vi "MOV and qTAV.vi"(0 "System no.":i32=1 min=1 max=4 step=1, 1 "Board":i32=1 min=1 max=5 step=1, 2 "Axes to move":string[](array[string]), 3 "Position values":dbl[](array[numeric]) format="%.6f", 4 "No.of digits":i16=4, 5 "error in":errorcluster, 7 "Polling\nCycle time, ms":u32=1, 9 "Wait before\nTAV?, ms":u32=1, 12 "Stop refnum":refnum<vi>) -> (14 "Analog value":dbl format="%.3f", 19 "error out":errorcluster)   [LabVIEW 2026]
doc: "Moves stage to absolute position (MOV.vi), waits for the specified axes to stop (General wait for movement to stop.vi) and queries TAV? (TAV?.vi). A wait time before the TAV? query can be defined. Define connected systems.vi must be run before running this VI. Requires Wait for axes to stop.vi, #5.vi, STA?.vi, #5_old.vi, ONT?.vi and Wait for hexapod system axes to stop.vi to be present.\n\nE-712: \nE-761: Board = 4. The output is the current voltage at the analog input line, with gain and offset."
panel:
  in  "Local stop":bool
  # "Moves stage to absolute position (MOV.vi), waits for the specified axes to stop (General wait for \nmovement to stop.vi) and queries TAV? (TAV?.vi). A wait time before the TAV? query can be defined. \n\"Define connected systems.vi\" must be run before running this vi. Requires \"Wait for axes to stop.vi\", \n\"#5.vi\",\"STA?.vi\", \"#5_old.vi\", \"ONT?.vi\" and \"Wait for hexapod system axes to stop.vi\" to be present."
  # "For MOV:"
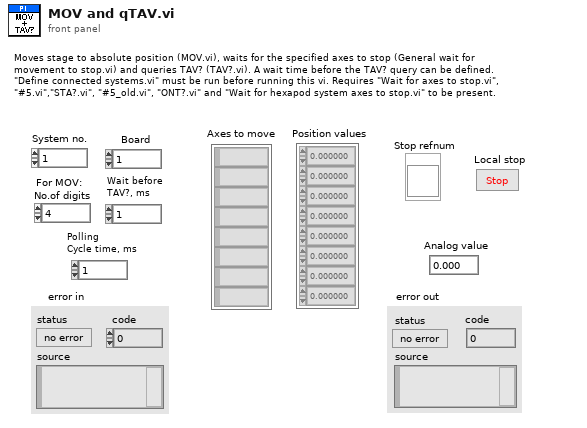
[diagram p1: front panel]
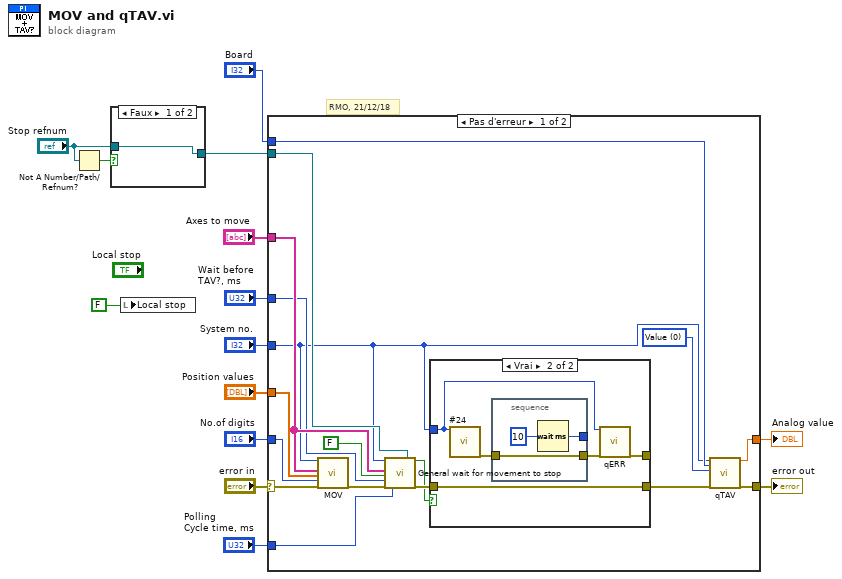
[diagram p0: block diagram]
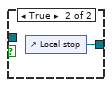
[diagram p2: hidden frame]
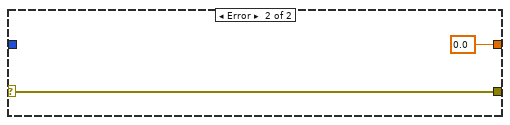
[diagram p4: hidden frame]
diagram:
  # "RMO, 21/12/18"
  n1 = Not A Number/Path/Refnum?(number/path/refnum="Stop refnum") -> (NaN/Path/Refnum?=w4:bool)
  n2 = case shown="Faux" w4 {
    tunnel: [w15 w16] -> w2
    tunnel: "Stop refnum" -> [w15 _]
    frame False {
    }
    frame True {
      n3 = control-ref of="Local stop"() -> (w16:refnum<vi>)
    }
  }
  n4 = local write "Local stop"(FALSE ("Finished")) -> ()
  n5 = case shown="Pas d'erreur" "error in" {
    selector: "error in" -> [w17 w43]
    tunnel: [w28 w43] -> w14
    tunnel: "No.of digits" -> [w32 _]
    tunnel: "System no." -> [w18 _]
    tunnel: "Axes to move" -> [w31 _]
    tunnel: "Position values" -> [w33 _]
    tunnel: "Board" -> [w29 _]
    tunnel: [w27 0.0 ("Analog value")] -> w8
    tunnel: "Polling\nCycle time, ms" -> [w26 _]
    tunnel: "Wait before\nTAV?, ms" -> [w25 _]
    tunnel: w2 -> [w20 _]
    frame No Error {
      w23 = u16 0 items=["Value", "Range", "Power unit"] ("Query")
      n6 = call "MOV.vi"("System no."=w18, "Axes to move"=w31, "Position values"=w33, "No.of digits"=w32, "error in"=w17) -> ("error out"=w30:errorcluster)  [unwired: 14 out]
      n7 = call "General wait for movement to stop.vi"("System no."=w18, "Axes to wait for"=w31, "All axes?"=FALSE, "Additional wait time, ms"=w25, "error in"=w30, "Polling cycle \ntime, ms"=w26, "Stop refnum"=w20) -> ("Stopped"=w19:bool, "error out"=w22:errorcluster)  [unwired: 1 in, 10 out]
      n8 = case shown="Vrai" w19 {
        tunnel: w22 -> [w34 w36]
        tunnel: [w34 w36] -> w21
        tunnel: w18 -> [_ w39]
        tunnel: [w34 w35] -> _
        frame False {
        }
        frame True {
          n9 = call "#24.vi"("System no."=w39) -> ("error out"=w38:errorcluster)  [unwired: 1 in, 17 out]
          n10 = stacked-sequence {
            tunnel: w38 -> [w41]
            tunnel: [w41] -> w37
            tunnel: [w40] -> _
            frame #0 {
              n11 = Wait (ms)(milliseconds to wait=u32 10) -> (millisecond timer value=w40:u32)
            }
          }
          n12 = call "qERR.vi"("System no."=w39, "error in"=w37) -> ("error out"=w35:errorcluster)  [unwired: 17 out]
        }
      }
      n13 = call "qTAV.vi"("System no."=w18, "Board"=w29, "Query"=w23, "error in"=w21) -> ("Analog value"=w27:dbl, "error out"=w28:errorcluster)  [unwired: 14 out]
    }
    frame Error {
    }
  }
  "error out" <- w14
  "Analog value" <- w8
